vi "Flush Data to Log File.vi"(8 "error in (no error)":errorcluster, 10 "data queue in":refnum<queue>, 11 "Logging Configuration":T1) -> (0 "error out":errorcluster)   [LabVIEW 2026, in "Logging.lvlib"]
doc: "Flush the data queue of any pending data and write it to the log file. Close the TDMS file reference."
uses:
  Logging.lvlib
  Logging Configuration.ctl
  controls/NotifierAndDataQueue.ctl
  controls/WaveformChartData.ctl
  Settings/Settings.lvlib
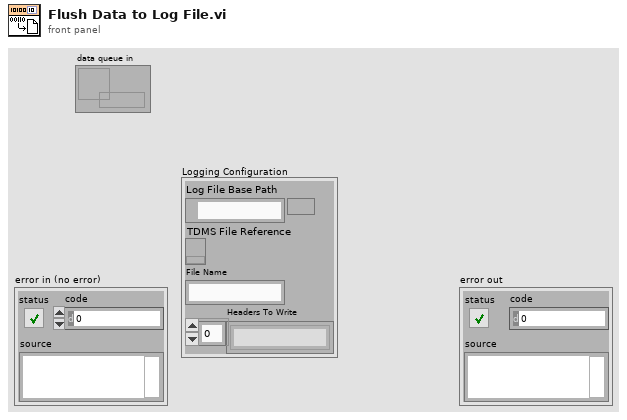
[diagram p1: front panel]
types:
  T1 = typedef "Logging.lvlib/Logging Configuration.ctl" = cluster{"Log File Base Path":path, "TDMS File Reference":refnum<k34>, "File Name":string, "Headers To Write":string[]}
  T2 = typedef "NotifierAndDataQueue.ctl" = cluster{"Ai0":dbl, "Ai1":dbl, "Ai2":dbl, "Ai3":dbl, "Ai4":dbl, "Ai5":dbl, "Ai6":dbl, "Ai7":dbl, "P0.0":bool, "P0.1":bool, "P0.2":bool, "P0.3":bool, "P0.4":bool, "P0.5":bool, "P0.6":bool, "P0.7":bool, "2D Numeric Data":dbl[][], "String 2":string, "String 1":string, "Waveform Chart Data":T3}
  T3 = typedef "Settings.lvlib/WaveformChartData.ctl" = cluster{"DUT Vacuum":dbl, "Motor RPM":dbl}
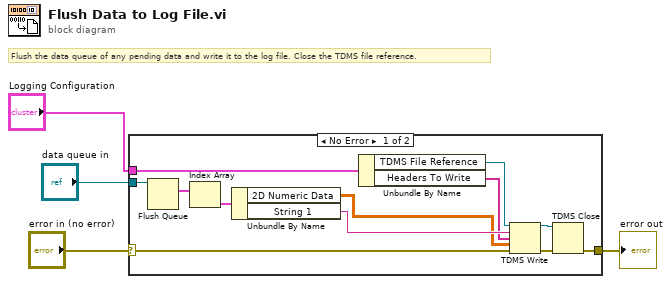
[diagram p0: block diagram]
diagram:
  # "Flush the data queue of any pending data and write it to the log file. Close the TDMS file reference."
  n1 = case shown="No Error" "error in (no error)" {
    selector: "error in (no error)" -> [w13 w17]
    tunnel: "Logging Configuration" -> [w15 _]
    tunnel: [w14 w17] -> w3
    tunnel: "data queue in" -> [w12 _]
    frame No Error {
      n2 = Flush Queue(queue=w12) -> (remaining elements=w10:T2[])  [unwired: 1 in, 2 out]
      n3 = Index Array(array=w10) -> (element=w9:T2)  [unwired: 1 in]
      n4 = Unbundle By Name(w9) -> ("2D Numeric Data"=w5:dbl[][], "String 1"=w7:string)
      n5 = Unbundle By Name(w15) -> ("TDMS File Reference"=w16:refnum<k34>, "Headers To Write"=w6:string[])
      n6 = TDMS Write(0:w16, 5:w7, 7:w6, 9:w5, 11:w13) -> (4:w8:refnum<k34>, 15:w11:errorcluster)  [unwired: 1 in, 2 out]
      n7 = TDMS Close(8:w11, 11:w8) -> (0:w14:errorcluster)  [unwired: 1 out]
    }
    frame Error {
    }
  }
  "error out" <- w3
